vi "CN Tab.vi"() -> ()   [LabVIEW 2014]
uses:
  Type'def/CN Product Ctr.ctl
  Type'def/CN Product1_4 Ctr.ctl
  Type'def/CN Product1_5 Ctr.ctl
panel:
  in  "Tab CN":enum32{"1/2", "1/3", "1/4", "1/5", "2/5", "3/5"}(tab)
  out "CN image2/2":T1
  out "CN image1/2":T1
  out "CN image3/3":T1
  out "CN image2/3":T1
  out "CN image1/3":T1
  out "CN image4/4":T2
  out "CN image3/4":T2
  out "CN image2/4":T2
  out "CN image1/4":T2
  out "CN image5/5":T3
  out "CN image4/5":T3
  out "CN image3/5":T3
  out "CN image2/5":T3
  out "CN image1/5":T3
  out "CN image5/5 2":T3
  out "CN image4/5 2":T3
  out "CN image3/5 2":T3
  out "CN image2/5 2":T3
  out "CN image1/5 2":T3
  out "CN image5/5 3":T3
  out "CN image4/5 3":T3
  out "CN image3/5 3":T3
  out "CN image2/5 3":T3
  out "CN image1/5 3":T3
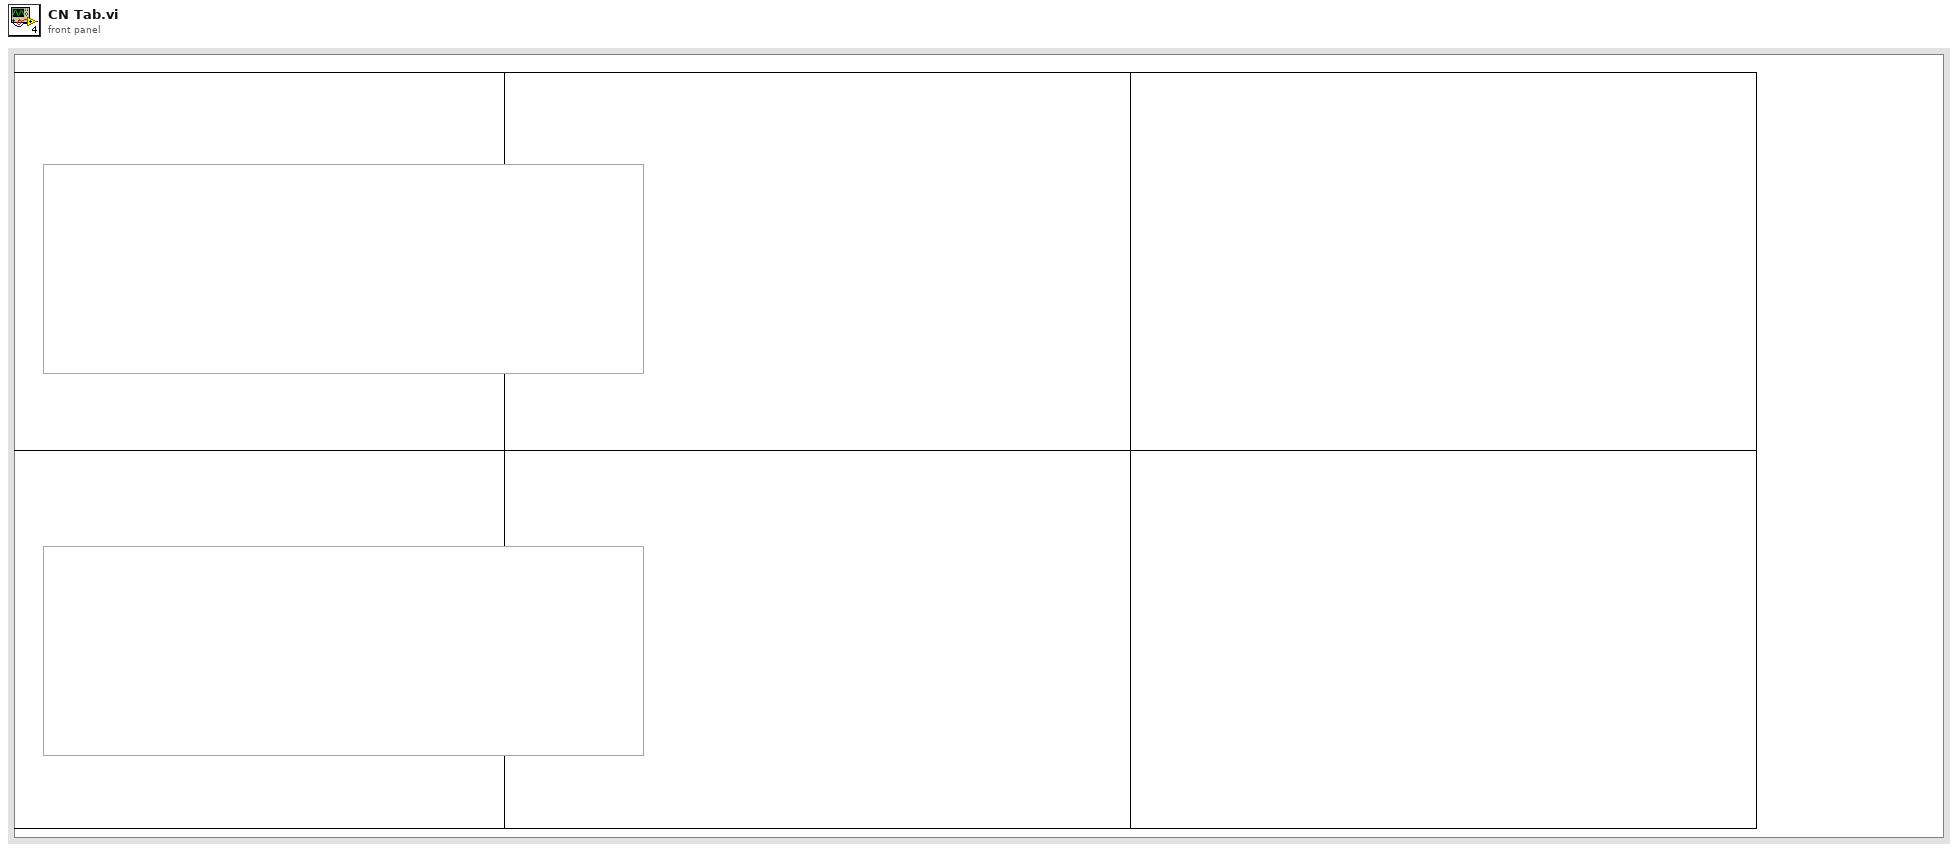
[diagram p1: front panel]
types:
  T1 = typedef "CN Product Ctr.ctl" = cluster{"2D Picture 3":picture, "Model":string, "Brand":string}
  T2 = typedef "CN Product1_4 Ctr.ctl" = cluster{"2D Picture 3":picture, "Model":string, "Brand":string}
  T3 = typedef "CN Product1_5 Ctr.ctl" = cluster{"2D Picture 3":picture, "Model":string, "Brand":string}
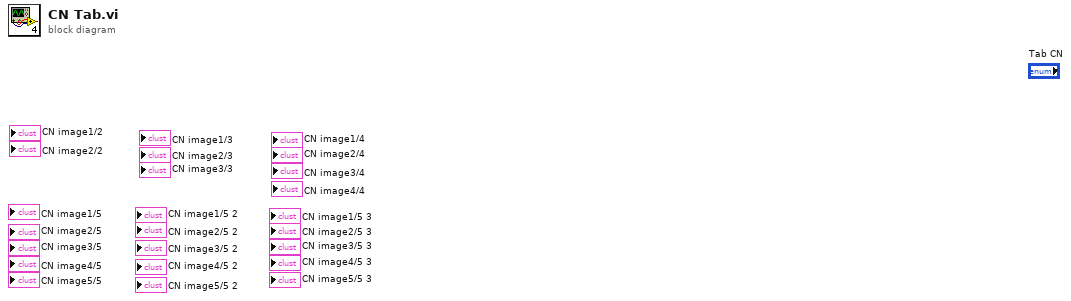
[diagram p0: block diagram]
diagram:
